vi "Test_Observe_ViewablePublication_OK.vi"(8 "error in (no error)":errorcluster, 11 "TestObservation In":refnum<class "TestPubSubRouting.lvclass">) -> (0 "error out":errorcluster, 3 "TestObservation Out":refnum<class "TestPubSubRouting.lvclass">)   [LabVIEW 2017, in "TestPubSubRouting.lvlib" / "TestPubSubRouting.lvclass"]
uses:
  TestPubSubRouting.lvclass
  Source/Framework/Mediator/Mediator/Mediator.lvclass
  C:/Git/mva-framework/Source/Framework/IMediator/IMediator/IMediator.lvclass
  PublishingViewable/PublishingViewable.lvclass
  C:/Git/mva-framework/Source/Framework/IObserver/IObserver/IObserver.lvclass
  C:/Git/mva-framework/Source/Framework/IViewable/IViewable/IViewable.lvclass
  gpm_packages/@cs/event-logger/Source/Composed Log/LoggerReference/LoggerReference.lvclass/LoggerReference.ctl
  Source/Framework/IObserver/IObserver/IObserver.lvclass/IObserver.ctl
  Source/Framework/IMediator/IMediator/IMediator.lvclass/IMediator.ctl
  Source/Framework/IViewModel/IViewModel/IViewModel.lvclass/IViewModel.ctl
  Source/Framework/IViewManager/IViewManager Messages/Launch Nested Views Msg/Launch Nested Views Msg.lvclass/Launch Nested Views Msg.ctl
  Source/Framework/IViewManager/IViewManager/IViewManager.lvclass/IViewManager.ctl
  <vilib>/ActorFramework/Message Enqueuer/Message Enqueuer.lvclass/Message Enqueuer.ctl
  ede1f806-c2ad-41f4-aa88-3ea56a4d09f1.vi
  ede1f806-c2ad-41f4-aa88-3ea56a4d09f1.vi/85c034b2-ac92-462b-8e95-3d1b84f0857b.vi
  Source/Framework/IObserver/IObserver/Configure Observer Logging.vi
  Source/Framework/IViewModel/IViewModel/Write Startup Model-View Configuration.vi
  Source/Framework/IMediator/IMediator/Configure Mediator.vi
  <vilib>/ActorFramework/Message Enqueuer/Enqueue.vi
  gpm_packages/@cs/event-logger/Source/Composed Log/LoggerReference/Return Aggregate Queues.vi
  gpm_packages/@cs/event-logger/Source/Composed Log/LoggerReference/Add Aggregate Log.vi
  ede1f806-c2ad-41f4-aa88-3ea56a4d09f1.vi/85c034b2-ac92-462b-8e95-3d1b84f0857b.vi/489b06a7-d78e-4ad4-8f96-f13fbf636d2b.vi
  Source/Framework/IViewManager/IViewManager Messages/Launch Nested Views Msg/Pack Launch Nested Views Msg.vi
  Source/Framework/IViewManager/IViewManager/Write Startup Launch Nested Views Msg.vi
  gpm_packages/@cs/event-logger/Source/Composed Log/LoggerReference/Send Add Sink.vi
  gpm_packages/@cs/event-logger/Source/Text File Sink/Text File Sink.lvclass
  C:/Git/mva-framework/gpm_packages/@cs/event-logger/Source/Composed Log/Log Sink/Log Sink.lvclass
  ObservingModel/ObservingModel.lvclass
  C:/Git/mva-framework/Source/Framework/IModel/IModel/IModel.lvclass
  ObservingViewModel/ObservingViewModel.lvclass
  C:/Git/mva-framework/Source/Framework/IViewModel/IViewModel/IViewModel.lvclass
  C:/Program Files (x86)/National Instruments/LabVIEW 2017/vi.lib/ActorFramework/Actor/Actor.lvclass
  Source/Framework/IViewModel/IViewModel/IViewModel.lvclass
  C:/Git/mva-framework/Source/Framework/IViewManager/IViewManager/IViewManager.lvclass
  <vilib>/ActorFramework/Stop Msg/Stop Msg.lvclass
  C:/Program Files (x86)/National Instruments/LabVIEW 2017/vi.lib/ActorFramework/Message/Message.lvclass
  gpm_packages/@cs/event-logger/Source/Composed Log/Application Logger/Launch Worker Loop.vi
  gpm_packages/@cs/event-logger/Source/Composed Log/LoggerReference/Initialize Logger Instance.vi
  <vilib>/ActorFramework/Message Priority Queue/Priority Enqueue.vi
  gpm_packages/@cs/event-logger/Source/Composed Log/LoggerReference/LoggerReference.lvclass
  Source/Framework/IMediator/IMediatorBusMonitor/IMediatorBusMonitor.lvclass
  gpm_packages/@cs/event-logger/Source/Composed Log/IErrorFormat/IErrorFormat.lvclass
  gpm_packages/@cs/event-logger/Source/Composed Log/Log Sink/Log Sink.lvclass
  Source/Framework/IViewable/IApplicationStyle/IApplicationStyle.lvclass
  Source/Framework/IViewManager/IViewManager Messages/Launch Nested Views Msg/Launch Nested Views Msg.lvclass
  <vilib>/ActorFramework/Actor/Actor.lvclass
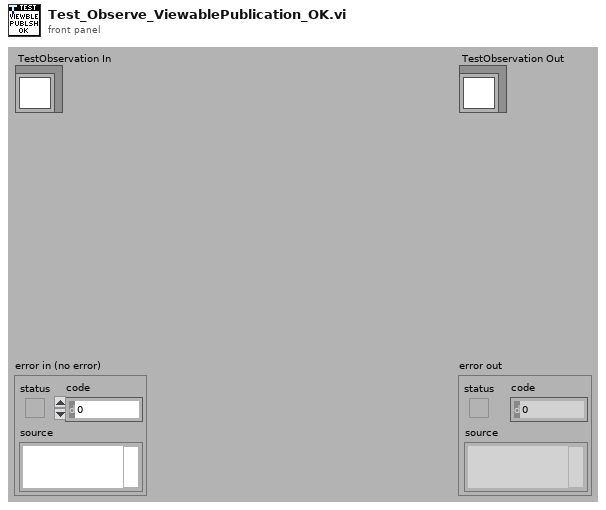
[diagram p1: front panel]
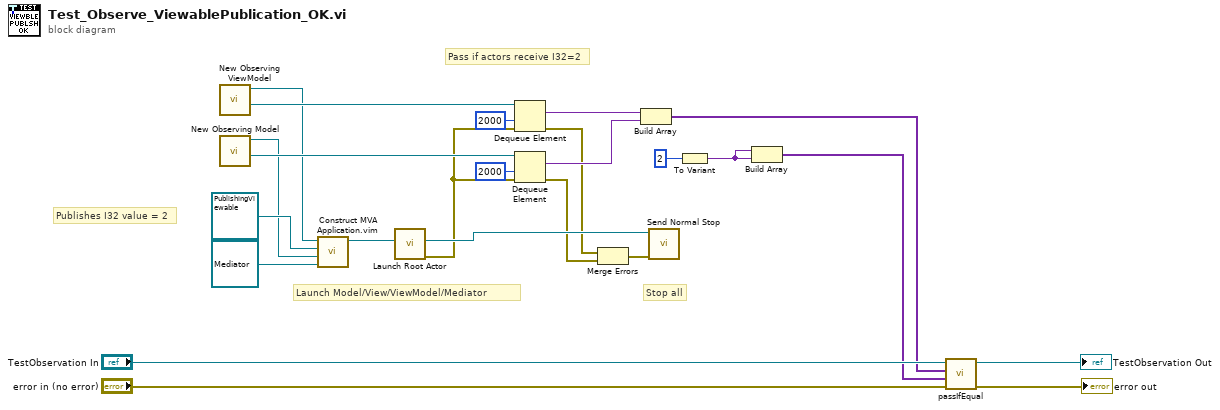
[diagram p0: block diagram]
diagram:
  # "Publishes I32 value = 2"
  # "Stop all"
  # "Launch Model/View/ViewModel/Mediator"
  # "Pass if actors receive I32=2"
  n1 = call "New Observing ViewModel.vi"() -> ("Test Reply Queue"=w10:refnum<queue>, "ObservingViewModel Out"=w5:refnum<class "ObservingViewModel.lvclass">)  [unwired: 10 in]
  n2 = call "New Observing Model.vi"() -> ("Test Reply Queue"=w13:refnum<queue>, "ObservingModel Out"=w6:refnum<class "ObservingModel.lvclass">)  [unwired: 10 in]
  n3 = call "Construct MVA Application.vim"("Mediator Type"=refnum<class "Mediator.lvclass"> refnum ("Mediator.lvlib:Mediator.lvclass"), "Model Type"=w6, "Startup View Configuration"=refnum<class "PublishingViewable.lvclass"> refnum ("PublishingViewable.lvclass"), "IViewModel In"=w5) -> ("IViewModel Out"=w19:refnum<class "ObservingViewModel.lvclass">)  [unwired: 7 in]
  n4 = call <vilib>:"Launch Root Actor.vi"("Actor"=w19) -> ("error out"=w9:errorcluster, "Actor's Enqueuer"=w17:refnum<class "Message Enqueuer.lvclass">)  [unwired: 9 in]
  n5 = Dequeue Element(queue=w10, timeout in ms (-1)=2000, error in (no error)=w9) -> (element=w3:variant, error out=w7:errorcluster)  [unwired: 2 out]
  n6 = Dequeue Element(queue=w13, timeout in ms (-1)=2000, error in (no error)=w9) -> (element=w15:variant, error out=w16:errorcluster)  [unwired: 2 out]
  n7 = Merge Errors(w7, w16) -> (w8:errorcluster)
  n8 = Build Array(w3, w15) -> (w4:variant[])
  n9 = call <vilib>:"Send Normal Stop.vi"("error in (no error)"=w8, "Message Enqueuer"=w17) -> ()  [unwired: 9 in, 1 out]
  n10 = To Variant(anything=2) -> (Variant=w1:variant)
  n11 = Build Array(w1, w1) -> (w2:variant[])
  n12 = call-dynamic "passIfEqual.vi"("error in (no error)"="error in (no error)", "y"=w2, "x"=w4, "TestCase in"="TestObservation In") -> ("error out"=→"error out":errorcluster, "TestCase out"=→"TestObservation Out":refnum<class "TestPubSubRouting.lvclass">)  [unwired: 6 in]
